vi "GCOMM Open.vi"(8 "error in":errorcluster, 11 "session in":T1) -> (0 "error out":errorcluster, 2 "idn string":string, 3 "session out":T1)   [LabVIEW 2013]
doc: "Opens generic COM port multiplexer."
uses:
  GCOMM Session.ctl
  GCOMM Signal.ctl
  GCOMM Virtual Channel.ctl
  GCOMM Logic State.ctl
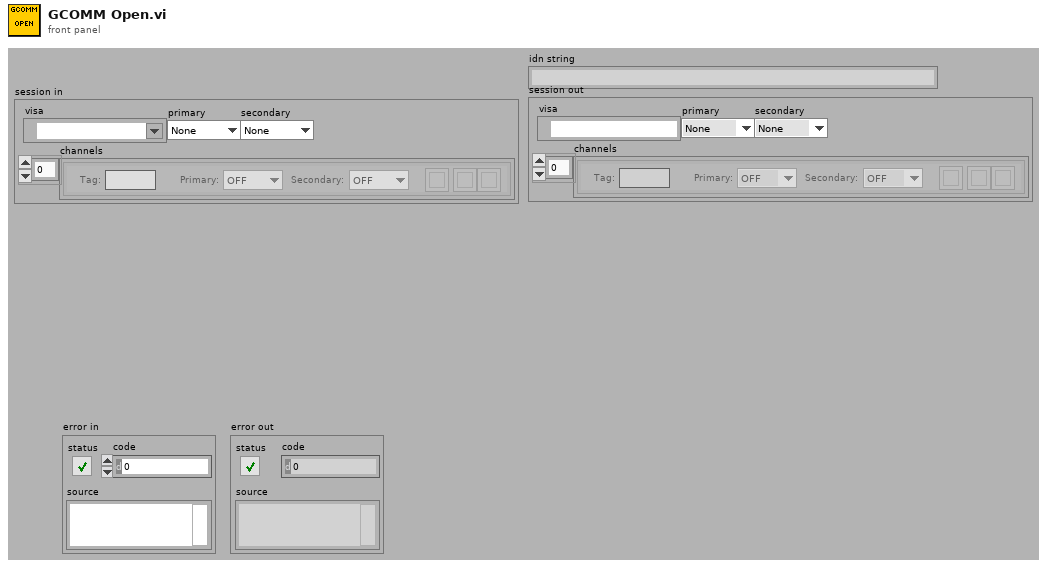
[diagram p1: front panel]
types:
  T1 = typedef "GCOMM Session.ctl" = cluster{"visa":refnum<visa-resource-name>, "primary":T2, "secondary":T2, "channels":T3[]}
  T2 = typedef "GCOMM Signal.ctl" = enum16{"None", "DTR", "RTS"}
  T3 = typedef "GCOMM Virtual Channel.ctl" = cluster{"Primary:":T4, "Secondary:":T4, "btn clr":bool, "btn up":bool, "btn down":bool, "Tag:":string}
  T4 = typedef "GCOMM Logic State.ctl" = enum16{"OFF", "ON"}
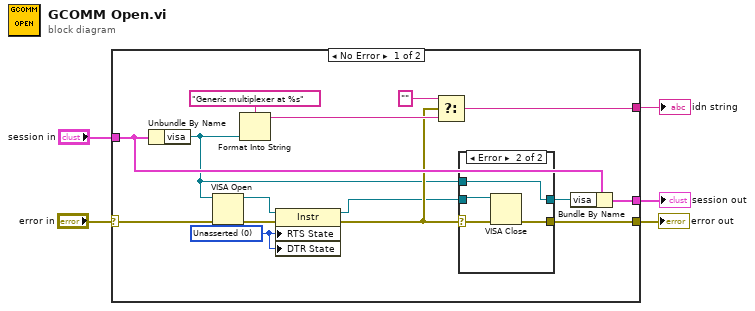
[diagram p0: block diagram]
diagram:
  n1 = case shown="No Error" "error in" {
    selector: "error in" -> [w14 w28]
    tunnel: [w9 w28] -> w5
    tunnel: [w13 _] -> w4
    tunnel: "session in" -> [w16 w27]
    tunnel: [w15 w27] -> w2
    frame No Error {
      w18 = i16 0 items=["Unknown"=-1, "Unasserted"=0, "Asserted"=1] ("Serial Settings:Modem Line Settings:Line RTS State")
      n2 = Unbundle By Name(w16) -> ("visa"=w6:refnum<visa-resource-name>)
      n3 = VISA Open(error in (no error)=w14, VISA resource name=w6) -> (VISA resource name=w19:refnum<visa-resource-name>, error out=w20:errorcluster)  [unwired: 3 in]
      n4 = Format Into String(format string="Generic multiplexer at %s", w6) -> (resulting string=w12:string)  [unwired: 2 in, 1 out]
      n5 = property class="Instr"(reference=w19, error in=w20, "RTS State"=w18, "DTR State"=w18) -> (reference out=w7:refnum<visa-resource-name>, error out=w10:errorcluster)
      n6 = Select(t="", s=w10, f=w12) -> (s? t:f=w13:string)
      n7 = case shown="Error" w10 {
        selector: w10 -> [w22 w26]
        tunnel: [w22 w25] -> w9
        tunnel: w7 -> [w21 w24]
        tunnel: [w21 w23] -> w8
        tunnel: w6 -> [_ w23]
        frame No Error {
        }
        frame Error {
          n8 = VISA Close(VISA resource name=w24, error in (no error)=w26) -> (error out=w25:errorcluster)
        }
      }
      n9 = Bundle By Name(cluster=w16, "visa"=w8) -> (w15:T1)
    }
    frame Error {
    }
  }
  "error out" <- w5
  "idn string" <- w4
  "session out" <- w2
